vi "Case Structures - Arithmetic Operations.vi"() -> ()   [LabVIEW 2016]
panel:
  in  "Case":i32=3
  out "O/P":dbl
  in  "I/P 2":dbl
  in  "I/P 1":dbl
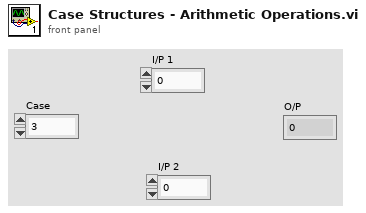
[diagram p1: front panel]
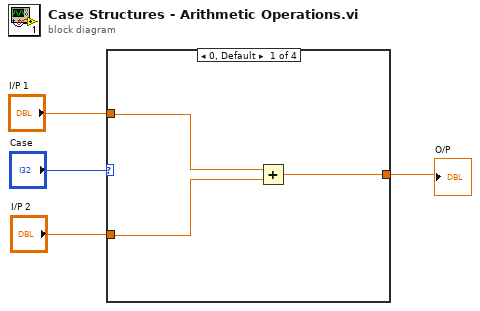
[diagram p0: block diagram]
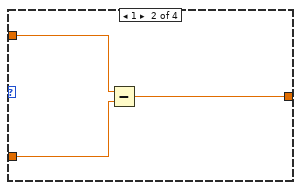
[diagram p2: hidden frame]
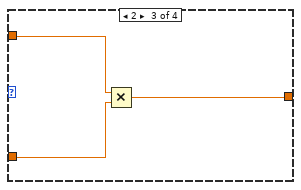
[diagram p3: hidden frame]
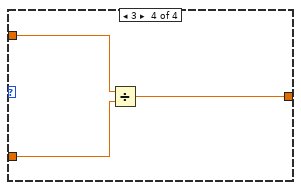
[diagram p4: hidden frame]
diagram:
  n1 = case shown="0, Default" "Case" {
    tunnel: "I/P 1" -> [w7 w10 w13 w15]
    tunnel: "I/P 2" -> [w6 w9 w12 w14]
    tunnel: [w5 w8 w11 w16] -> w2
    frame 0, Default {
      n2 = Add(x=w7, y=w6) -> (x+y=w5:dbl)
    }
    frame 1 {
      n3 = Subtract(x=w10, y=w9) -> (x-y=w8:dbl)
    }
    frame 2 {
      n4 = Multiply(x=w13, y=w12) -> (x*y=w11:dbl)
    }
    frame 3 {
      n5 = Divide(x=w15, y=w14) -> (x/y=w16:dbl)
    }
  }
  "O/P" <- w2
